vi "Strip Quoted String.vi"(8 "error in (no error)":errorcluster, 10 "Text":string, 11 "ProtoParser in":refnum<class "ProtoParser.lvclass">) -> (0 "error out":errorcluster, 1 "String Contents":string, 2 "Remaining":string, 3 "ProtoParser out":refnum<class "ProtoParser.lvclass">)   [LabVIEW 2020, in "LV-Protoc.lvlib" / "ProtoParser.lvclass"]
uses:
  ProtoParser.lvclass
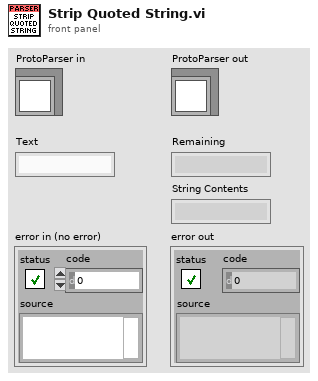
[diagram p1: front panel]
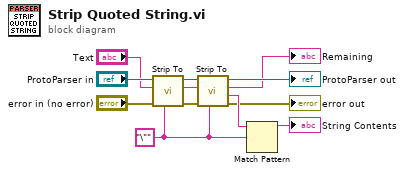
[diagram p0: block diagram]
diagram:
  w8 = "\"" ("End")
  n1 = call "Strip To.vi"("End"=w8, "error in (no error)"="error in (no error)", "String"="Text", "ProtoParser in"="ProtoParser in") -> ("error out"=w11:errorcluster, "Remaining"=w9:string, "ProtoParser out"=w10:refnum<class "ProtoParser.lvclass">)  [unwired: 4 in, 1 out]
  n2 = call "Strip To.vi"("End"=w8, "error in (no error)"=w11, "String"=w9, "ProtoParser in"=w10) -> ("error out"=→"error out":errorcluster, "Portion"=w7:string, "Remaining"=→"Remaining":string, "ProtoParser out"=→"ProtoParser out":refnum<class "ProtoParser.lvclass">)  [unwired: 4 in]
  n3 = Match Pattern(string=w7, regular expression=w8) -> (before substring=→"String Contents":string)  [unwired: 1 in, 3 out]
